vi "ExtractINIInfo.vi"(11 "INI File Path":path) -> (0 "INI File Name Without Extension":string, 1 "INI File Name":string, 2 "Instrument name":string, 3 "Module Name":string, 4 "Visualization VI Path":path, 5 "Module.INI File Name":string, 6 "Instrument Class Path":path)   [LabVIEW 2018]
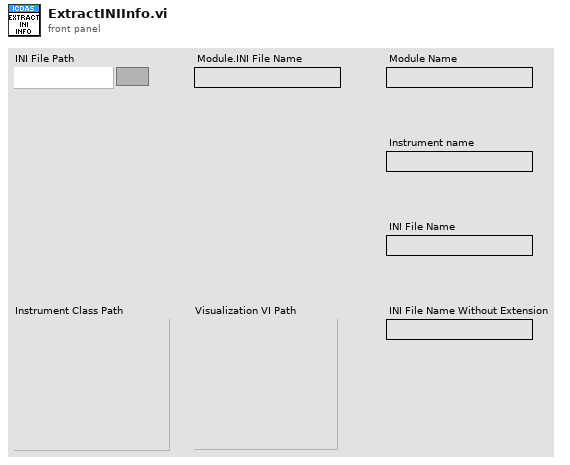
[diagram p1: front panel]
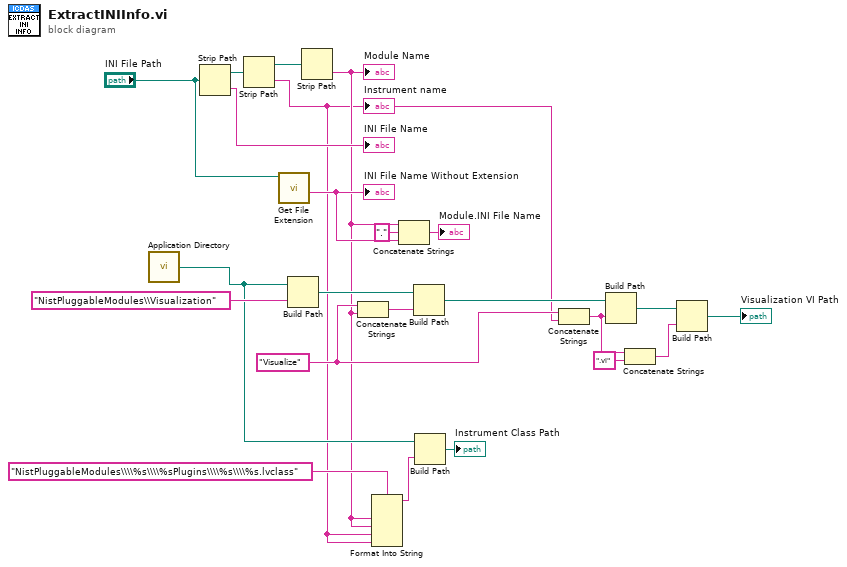
[diagram p0: block diagram]
diagram:
  w12 = "Visualize" ("string")
  n1 = call <vilib>:"Application Directory.vi"() -> ("Application Directory"=w5:path)
  n2 = Strip Path(path="INI File Path") -> (stripped path=w22:path, name=→"INI File Name":string)
  n3 = Strip Path(path=w22) -> (stripped path=w23:path, name=w3:string)
  "Instrument name" <- w3
  n4 = call <vilib>:"Get File Extension.vi"("file"="INI File Path") -> ("filename without extension"=w16:string)  [unwired: 6 in, 4 out]
  "INI File Name Without Extension" <- w16
  n5 = Build Path(base path=w5, name or relative path="NistPluggableModules\\Visualization") -> (appended path=w15:path)
  n6 = Strip Path(path=w23) -> (name=w4:string)  [unwired: 1 out]
  "Module Name" <- w4
  n7 = Concatenate Strings(w12, w4) -> (w13:string)
  n8 = Format Into String(format string="NistPluggableModules\\\\%s\\\\%sPlugins\\\\%s\\\\%s.lvclass" ("name or relative path"), w4, w4, w3, w3) -> (resulting string=w2:string)  [unwired: 2 in, 1 out]
  n9 = Concatenate Strings(w4, "." ("string"), w16) -> (→"Module.INI File Name":string)
  n10 = Build Path(base path=w15, name or relative path=w13) -> (appended path=w14:path)
  n11 = Build Path(base path=w5, name or relative path=w2) -> (appended path=→"Instrument Class Path":path)
  n12 = Concatenate Strings(w12, w3) -> (w9:string)
  n13 = Build Path(base path=w14, name or relative path=w9) -> (appended path=w11:path)
  n14 = Concatenate Strings(w9, ".vi" ("string")) -> (w10:string)
  n15 = Build Path(base path=w11, name or relative path=w10) -> (appended path=→"Visualization VI Path":path)
